vi "Try2_subVI.vi"(8 "error in (no error)":errorcluster, 9 "file path (dialog if empty)":path, 11 "connection ID":refnum<k5>) -> (0 "error out":errorcluster, 1 "data out":string, 3 "connection ID out":refnum<k5>)   [LabVIEW 2011]
uses:
  <vilib>/Utility/file.llb/Read From Spreadsheet File (DBL).vi
panel:
  out "data string":string
  in  "width (-)":i16
  in  "number":i32
  out "decimal integer string":string
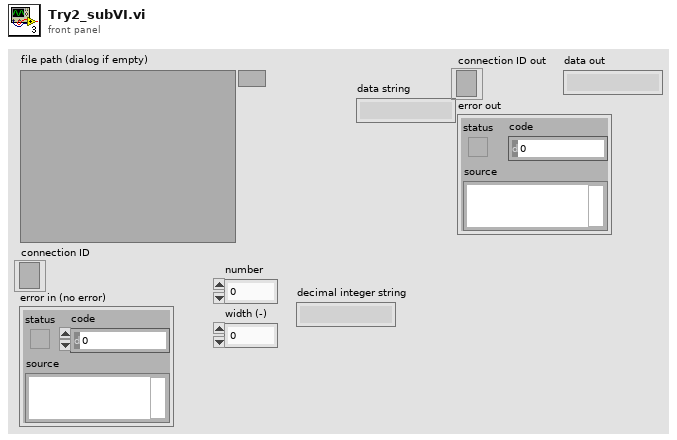
[diagram p1: front panel]
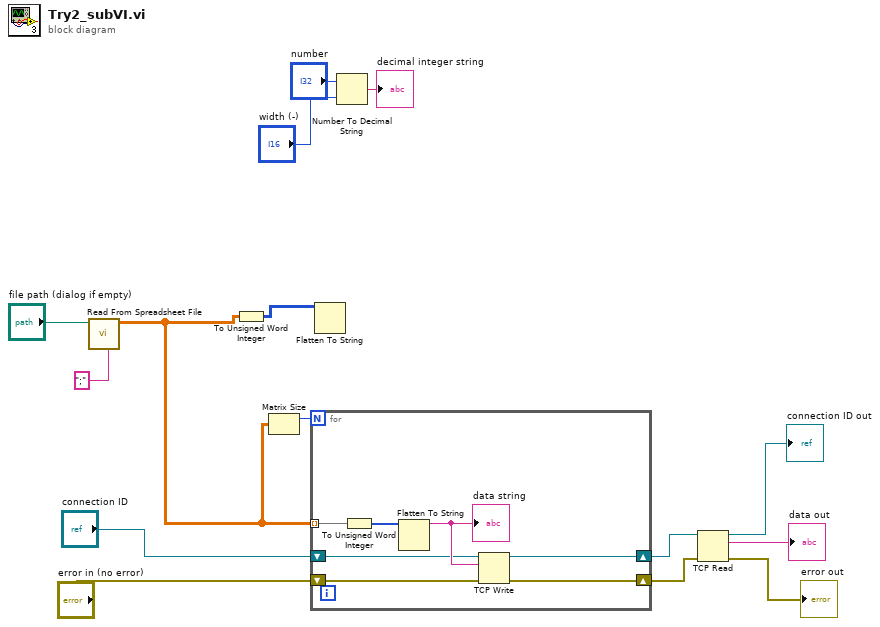
[diagram p0: block diagram]
diagram:
  n1 = call-poly <vilib>:"Read From Spreadsheet File.vi"("delimiter (\\t)"=";" ("delimiter (\\t)"), "file path (dialog if empty)"="file path (dialog if empty)") -> ("all rows"=w2:dbl[][])  [unwired: 5 in, 4 out]
  n2 = To Unsigned Word Integer(number=w2) -> (unsigned 16bit integer=w1:u16[][])
  n3 = Matrix Size(0:w2) -> (1:w10:i32)  [unwired: 1 out]
  n4 = for {
    N: w10 -> [_]
    tunnel: w2 -> [w22] mode=indexing
    shift-right: [w17] -> w7
    shift-left: "connection ID" -> [w19]
    shift-right: [w16] -> w6
    shift-left: "error in (no error)" -> [w18]
    n5 = To Unsigned Word Integer(number=w22) -> (unsigned 16bit integer=w21:u16[])
    n6 = Flatten To String(anything=w21) -> (data string=w20:string)  [unwired: 3 in, 2 out]
    "data string" <- w20
    n7 = TCP Write(connection ID=w19, data in=w20, error in (no error)=w18) -> (connection ID out=w17:refnum<k5>, error out=w16:errorcluster)  [unwired: 1 in, 1 out]
  }
  n8 = Flatten To String(anything=w1) -> ()  [unwired: 3 in, 3 out]
  n9 = Number To Decimal String(number="number", width (-)="width (-)") -> (decimal integer string=→"decimal integer string":string)
  n10 = TCP Read(connection ID=w7, error in (no error)=w6) -> (connection ID out=→"connection ID out":refnum<k5>, data out=→"data out":string, error out=→"error out":errorcluster)  [unwired: 3 in]
